vi "Read LPS Barometer.vi"(8 "error in (no error)":errorcluster, 11 "LINX-SenseHat in":refnum<class "LINX-SenseHat.lvclass">) -> (0 "error out":errorcluster, 2 "LPS25H Readings":T1, 3 "LINX-SenseHat out":refnum<class "LINX-SenseHat.lvclass">)   [LabVIEW 2020, in "LINX-SenseHat.lvclass"]
doc: "Reads temperature/pressure/altitude data from the LPS25H sensor on the Sense Hat."
uses:
  LINX-SenseHat.lvclass
  Barometer Readings.ctl
  LINX-SenseHat.lvclass/LINX-SenseHat.ctl
  LPS Barometric Pressure/LPS Barometric Pressure Sensor.lvclass
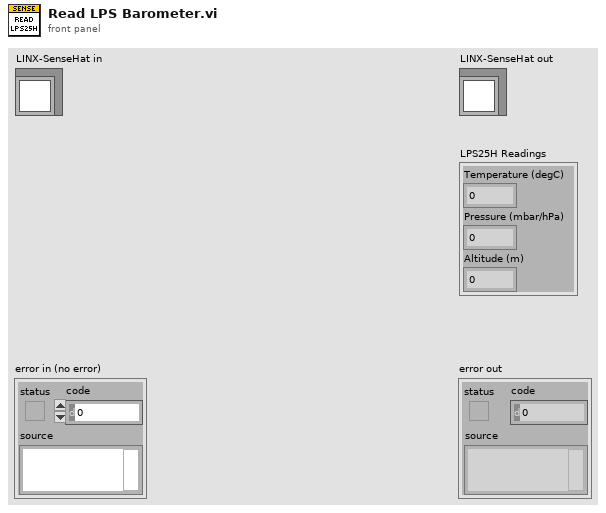
[diagram p1: front panel]
types:
  T1 = typedef "LINX-SenseHat.lvclass/Barometer Readings.ctl" = cluster{"Temperature (degC)":dbl, "Pressure (mbar/hPa)":dbl, "Altitude (m)":dbl}
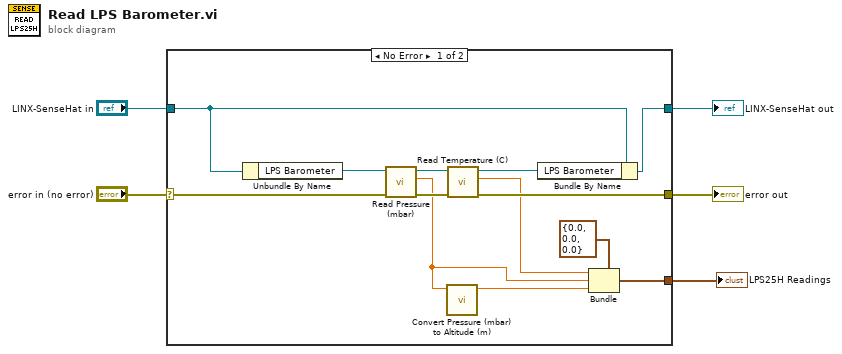
[diagram p0: block diagram]
diagram:
  n1 = case shown="No Error" "error in (no error)" {
    selector: "error in (no error)" -> [w15 w20]
    tunnel: [w14 w20] -> w4
    tunnel: [w6 w19] -> w2
    tunnel: "LINX-SenseHat in" -> [w7 w19]
    tunnel: [w9 _] -> w1
    frame No Error {
      n2 = Unbundle By Name(w7) -> ("LPS Barometer"=w18:refnum<class "LPS Barometric Pressure Sensor.lvclass">)
      n3 = call "Read Pressure (mbar).vi"("error in (no error)"=w15, "LPS Barometric Pressure Sensor in"=w18) -> ("error out"=w16:errorcluster, "Pressure (mbar/hPa)"=w12:dbl, "LPS Barometric Pressure Sensor out"=w17:refnum<class "LPS Barometric Pressure Sensor.lvclass">)  [unwired: 7 in]
      n4 = call "Convert Pressure (mbar) to Altitude (m).vi"("Pressure (mbar)"=w12) -> ("Altitude (m)"=w11:dbl)  [unwired: 10 in]
      n5 = call "Read Temperature (C).vi"("error in (no error)"=w16, "LPS Barometric Pressure Sensor in"=w17) -> ("error out"=w14:errorcluster, "Temperature (degC)"=w13:dbl, "LPS Barometric Pressure Sensor out"=w8:refnum<class "LPS Barometric Pressure Sensor.lvclass">)  [unwired: 7 in]
      n6 = Bundle By Name(cluster=w7, "LPS Barometer"=w8) -> (w6:refnum<class "LINX-SenseHat.lvclass">)
      n7 = Bundle(cluster=T1 {"Temperature (degC)"=0.0, "Pressure (mbar/hPa)"=0.0, "Altitude (m)"=0.0}, "Temperature (degC)"=w13, "Pressure (mbar/hPa)"=w12, "Altitude (m)"=w11) -> (w9:T1)
    }
    frame Error {
    }
  }
  "error out" <- w4
  "LINX-SenseHat out" <- w2
  "LPS25H Readings" <- w1
